vi "yc calculator.vi"(9 "Z":dbl, 10 "Y":dbl, 11 "X":dbl) -> (2 "yc":dbl)   [LabVIEW 2016, in "AMS TS3472 Light Sensor.lvlib" / "AMS TCS3472.lvclass"]
uses:
  AMS TCS3472.lvclass
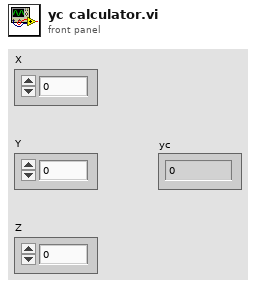
[diagram p1: front panel]
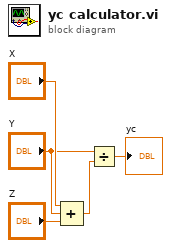
[diagram p0: block diagram]
diagram:
  n1 = Compound Arithmetic op=ADD("X", "Y", "Z") -> (w3:dbl)
  n2 = Divide(x="Y", y=w3) -> (x/y=→"yc":dbl)
